vi "Acquisition Message Loop.vi"(8 "error in (no error)":errorcluster, 9 "Data Queue":refnum<queue>, 10 "Data Notifier":refnum<notifier>, 11 "Message Queues":T1) -> (0 "error out":errorcluster)   [LabVIEW 2014, in "Flicker.lvlib" / "Flicker Acquisition.lvlib"]
doc: "Message loop for handling messages pertaining to the acquisition of data from the hardware."
uses:
  Flicker Acquisition.lvlib
  support/Message Queue/All Message Queues.ctl
  support/Message Queue/Message Cluster.ctl
  Hardware Configuration.ctl
  Signal Type.ctl
  support/Message Queue/Enqueue Message (Single).vi
  <vilib>/Utility/error.llb/Error Cluster From Error Code.vi
  <vilib>/ErrorRing/Error Ring.xnode
  support/Message Queue/Flicker Message Queue.lvlib
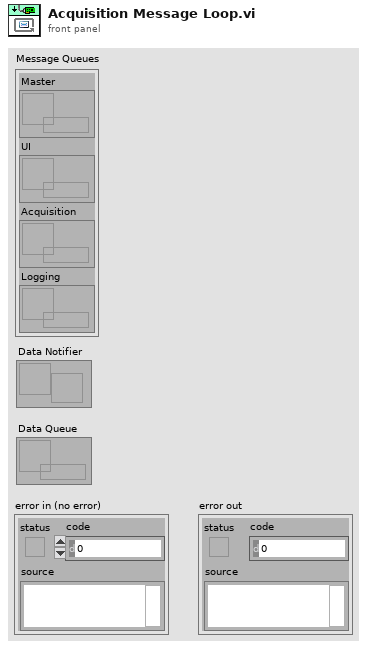
[diagram p1: front panel]
types:
  T1 = typedef "Flicker.lvlib/Flicker Message Queue.lvlib/All Message Queues.ctl" = cluster{"Master":refnum<queue>, "UI":refnum<queue>, "Acquisition":refnum<queue>, "Logging":refnum<queue>}
  T2 = typedef "Flicker.lvlib/Flicker Acquisition.lvlib/Hardware Configuration.ctl" = cluster{"DAQmx Task Name":refnum<k21>, "HW Refnum <Replace Me>":string, "Signal Type <Replace Me>":T3}
  T3 = typedef "Flicker.lvlib/Flicker Acquisition.lvlib/Signal Type.ctl" = enum16{"Sine Wave", "Square with Noise"}
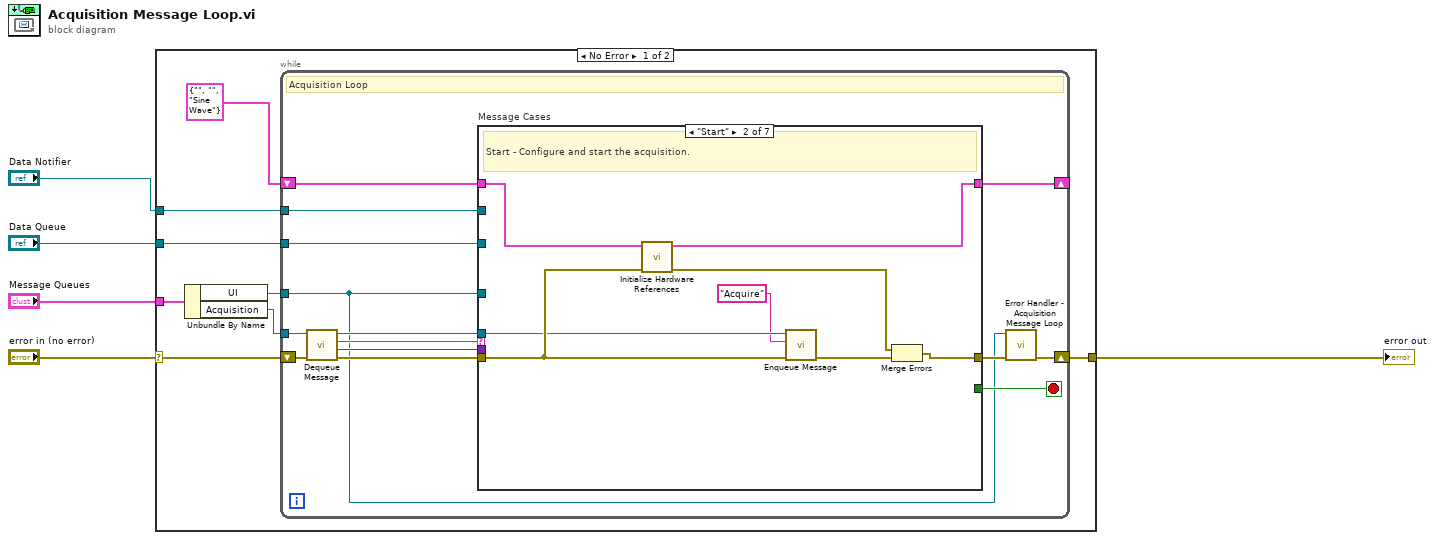
[diagram p0: block diagram]
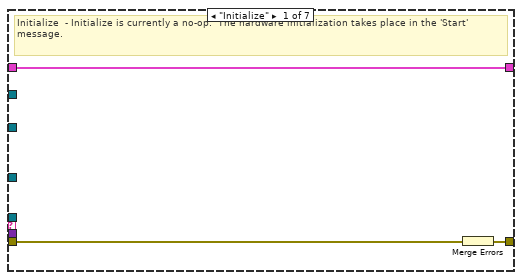
[diagram p2: hidden frame]
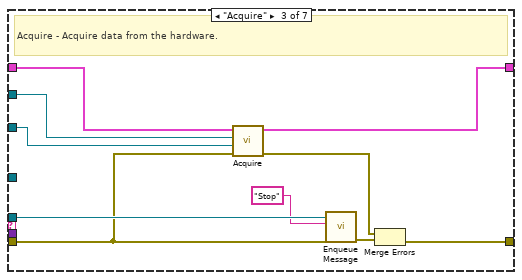
[diagram p3: hidden frame]
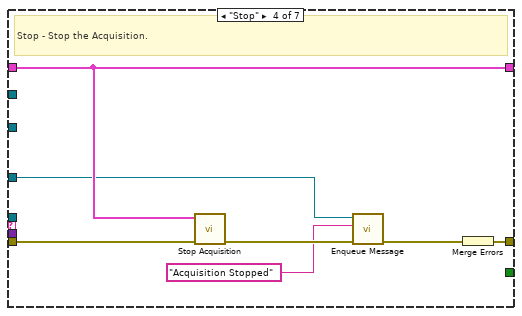
[diagram p4: hidden frame]
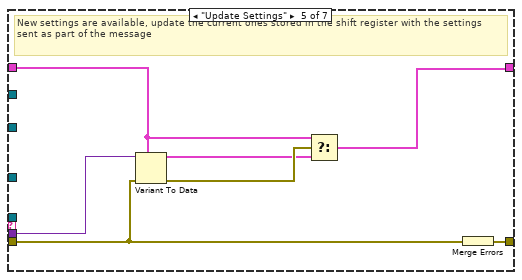
[diagram p5: hidden frame]
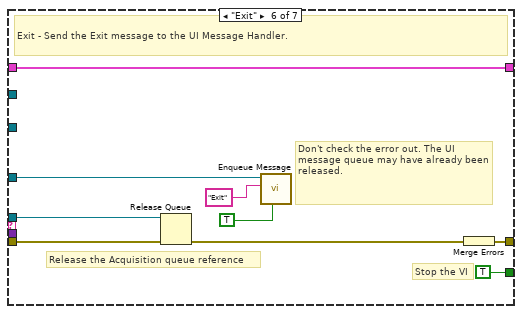
[diagram p6: hidden frame]
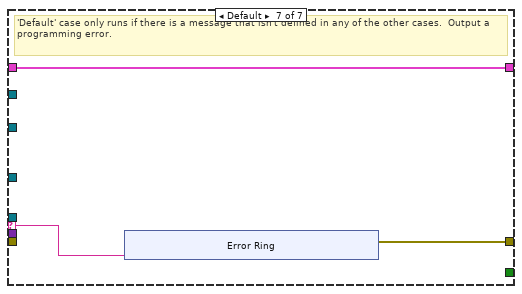
[diagram p7: hidden frame]
diagram:
  n1 = case shown="No Error" "error in (no error)" {
    selector: "error in (no error)" -> [w9 w82]
    tunnel: "Message Queues" -> [w13 _]
    tunnel: [w11 w82] -> w4
    tunnel: "Data Notifier" -> [w7 _]
    tunnel: "Data Queue" -> [w6 _]
    frame No Error {
      n2 = Unbundle By Name(w13) -> ("UI"=w8:refnum<queue>, "Acquisition"=w12:refnum<queue>)
      n3 = while {
        tunnel: w12 -> [w20]
        shift-right: [w26] -> _
        shift-left: T2 {"DAQmx Task Name"="", "HW Refnum <Replace Me>"="", "Signal Type <Replace Me>"=enum."Sine Wave"} ("Data Cluster") -> [w27]
        shift-right: [w17] -> w11
        shift-left: w9 -> [w24]
        tunnel: w8 -> [w14]
        tunnel: w7 -> [w19]
        tunnel: w6 -> [w18]
        stop <- w25 stop-if-true
        # "Acquisition Loop"
        n4 = call "Dequeue Message.vi"("error in (no error)"=w24, "Message Queue"=w20) -> ("error out"=w23:errorcluster, "Message Data"=w21:variant, "Message"=w22:string, "dup Message Queue"=w15:refnum<queue>)  [unwired: 6 in]
        n5 = case "Message Cases" shown="\"Start\"" w22 {
          selector: w22 -> [_ _ _ _ _ _ w72]
          tunnel: w15 -> [_ w35 w47 _ _ w63 _]
          tunnel: w23 -> [w29 w36 w46 w54 w56 w67 _]
          tunnel: [w30 w38 w48 w55 w62 w70 w73] -> w16
          tunnel: w27 -> [w28 w37 w44 w52 w58 w69 w74]
          tunnel: [w28 w34 w45 w52 w57 w69 w74] -> w26
          tunnel: [_ _ _ _ _ TRUE _] -> w25
          tunnel: w21 -> [_ _ _ _ w61 _ _]
          tunnel: w14 -> [_ _ _ w51 _ w68 _]
          tunnel: w19 -> [_ _ w43 _ _ _ _]
          tunnel: w18 -> [_ _ w42 _ _ _ _]
          frame "Initialize" {
            # "Initialize  - Initialize is currently a no-op.  The hardware initialization takes place in the 'Start' message."
            n6 = Merge Errors(w29) -> (w30:errorcluster)
          }
          frame "Start" {
            # "Start - Configure and start the acquisition."
            n7 = call "Initialize Hardware References.vi"("error in (no error)"=w36, "Hardware Resources in"=w37) -> ("error out"=w31:errorcluster, "Hardware Resources out"=w34:T2)  [unwired: 8 in]
            n8 = call-poly "Enqueue Message.vi"("error in (no error)"=w36, "Message"="Acquire", "Message Queue"=w35) -> ("error out"=w33:errorcluster)  [unwired: 7 in, 1 out]
            n9 = Merge Errors(w31, w33) -> (w38:errorcluster)
          }
          frame "Acquire" {
            # "Acquire - Acquire data from the hardware."
            n10 = call "Acquire.vi"("error in (no error)"=w46, "Data Queue"=w42, "Data Notifier"=w43, "Hardware Resources in"=w44) -> ("error out"=w39:errorcluster, "Hardware Resources out"=w45:T2)  [unwired: 6 in]
            n11 = call-poly "Enqueue Message.vi"("error in (no error)"=w46, "Message"="Stop", "Message Queue"=w47) -> ("error out"=w40:errorcluster)  [unwired: 7 in, 1 out]
            n12 = Merge Errors(w39, w40) -> (w48:errorcluster)
          }
          frame "Stop" {
            # "Stop - Stop the Acquisition."
            n13 = call "Stop Acquisition.vi"("error in (no error)"=w54, "Hardware Resources in"=w52) -> ("error out"=w50:errorcluster)  [unwired: 9 in]
            n14 = call-poly "Enqueue Message.vi"("error in (no error)"=w50, "Message"="Acquisition Stopped", "Message Queue"=w51) -> ("error out"=w53:errorcluster)  [unwired: 7 in, 1 out]
            n15 = Merge Errors(w53) -> (w55:errorcluster)
          }
          frame "Update Settings" {
            # "New settings are available, update the current ones stored in the shift register with the settings sent as part of the message"
            n16 = Variant To Data(error in=w56, type=w58, Variant=w61) -> (data=w59:T2, error out=w60:errorcluster)
            n17 = Select(t=w58, s=w60, f=w59) -> (s? t:f=w57:T2)
            n18 = Merge Errors(w56) -> (w62:errorcluster)
          }
          frame "Exit" {
            # "Don't check the error out. The UI message queue may have already been released."
            # "Release the Acquisition queue reference"
            # "Stop the VI"
            # "Exit - Send the Exit message to the UI Message Handler."
            n19 = Release Queue(queue=w63, error in (no error)=w67) -> (error out=w64:errorcluster)  [unwired: 1 in, 2 out]
            n20 = call-poly "Enqueue Message.vi"("Priority Message? (F)"=TRUE, "Message"="Exit", "Message Queue"=w68) -> ()  [unwired: 7 in, 2 out]
            n21 = Merge Errors(w64) -> (w70:errorcluster)
          }
          frame Default {
            # "'Default' case only runs if there is a message that isn't defined in any of the other cases.  Output a programming error."
            n22 = xnode "Error Ring"("parameter 0"=w72) -> ("error out"=w73:errorcluster)
          }
        }
        n23 = call "Error Handler - Acquisition Message Loop.vi"("error in (no error)"=w16, "Message Queue"=w14) -> ("dup error in"=w17:errorcluster)  [unwired: 8 in, 1 out]
      }
    }
    frame Error {
    }
  }
  "error out" <- w4
